vi "(SubVI) Pearson Correlation Coefficient r^2_YCC.vi"(6 "best fit Data":dbl[](array[numeric]), 7 "Data":dbl[](array[numeric])) -> (2 "r^2":dbl, 3 "r":dbl)   [LabVIEW 2014]
uses:
  <vilib>/Analysis/NI_AALBase.lvlib
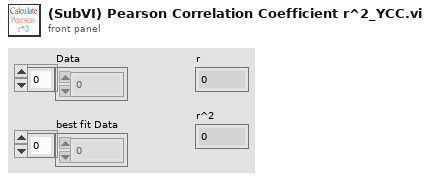
[diagram p1: front panel]
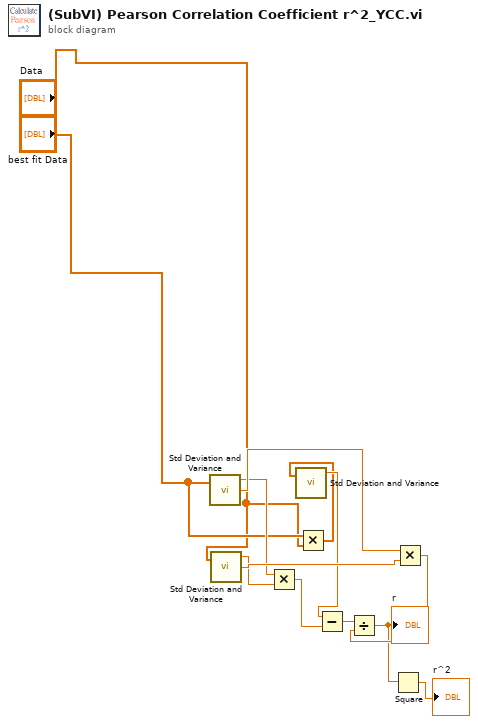
[diagram p0: block diagram]
diagram:
  n1 = call <vilib>:"Std Deviation and Variance.vi"("X"="best fit Data") -> ("mean"=w4:dbl, "standard deviation"=w9:dbl)  [unwired: 1 in, 1 out]
  n2 = call <vilib>:"Std Deviation and Variance.vi"("X"="Data") -> ("mean"=w5:dbl, "standard deviation"=w10:dbl)  [unwired: 1 in, 1 out]
  n3 = Multiply(x=w4, y=w5) -> (x*y=w7:dbl)
  n4 = Multiply(x="best fit Data", y="Data") -> (x*y=w3:dbl[])
  n5 = call <vilib>:"Std Deviation and Variance.vi"("X"=w3) -> ("mean"=w6:dbl)  [unwired: 1 in, 2 out]
  n6 = Subtract(x=w6, y=w7) -> (x-y=w8:dbl)
  n7 = Multiply(x=w9, y=w10) -> (x*y=w13:dbl)
  n8 = Divide(x=w8, y=w13) -> (x/y=w11:dbl)
  "r" <- w11
  n9 = Square(x=w11) -> (x^2=→"r^2":dbl)
